vi "testGetCmdUserEventInstance.vi"(8 "error in (no error)":errorcluster) -> (0 "error out":errorcluster)   [LabVIEW 2018]
doc: "Test the getCmdUserEventInstance.vi."
uses:
  src/TcpServer/TcpServer.lvclass
  src/TcpServer/typedef/packetConnIDTypeDef.ctl
  <vilib>/addons/_JKI Toolkits/Caraya/classes/Assert/Assert Equal Type_Variant.vi
  <vilib>/addons/_JKI Toolkits/Caraya/classes/Test/Test.lvclass
  <vilib>/addons/_JKI Toolkits/Caraya/classes/Assert/Assert.lvclass
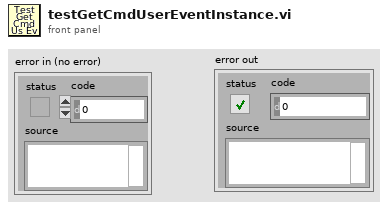
[diagram p1: front panel]
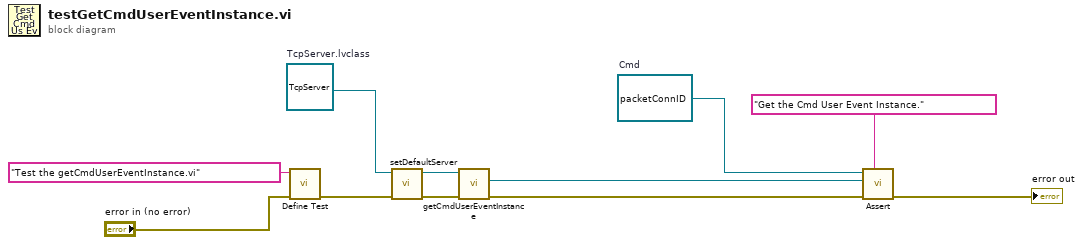
[diagram p0: block diagram]
diagram:
  w1 = refnum<user-event> refnum  # Cmd
  w8 = refnum<class "TcpServer.lvclass"> refnum  # TcpServer.lvclass
  n1 = call <vilib>:"Define Test.vi"("error in (no error)"="error in (no error)", "Label (VI Title)"="Test the getCmdUserEventInstance.vi") -> ("error out"=w10:errorcluster)  [unwired: 9 in]
  n2 = call "setDefaultServer.vi"("error in (no error)"=w10, "TcpServer.lvclass"=w8) -> ("error out"=w5:errorcluster, "tcpServer out"=w6:refnum<class "TcpServer.lvclass">)  [unwired: 8 in]
  n3 = call "getCmdUserEventInstance.vi"("error in (no error)"=w5, "tcpServer in"=w6) -> ("error out"=w3:errorcluster, "Cmd"=w4:refnum<user-event>)  [unwired: 7 in, 1 out]
  n4 = call-poly <vilib>:"Assert.vi"("Label"="Get the Cmd User Event Instance.", "error in (no error)"=w3, "Y"=w4, "X"=w1) -> ("error out"=→"error out":errorcluster)  [unwired: 7 in]
